vi "TF_Encoder2Position.vi"(2 "Counter Value":i32, 4 "Offset":dbl) -> (5 "Position [deg]":dbl format="%#_13g")   [LabVIEW 2019]
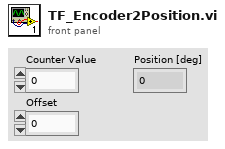
[diagram p1: front panel]
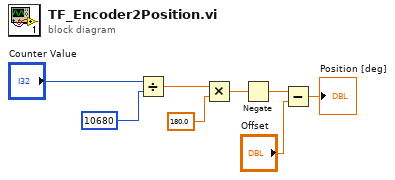
[diagram p0: block diagram]
diagram:
  n1 = Divide(x="Counter Value", y=10680) -> (x/y=w7:dbl)
  n2 = Multiply(x=w7, y=180.0) -> (x*y=w5:dbl)
  n3 = Negate(x=w5) -> (-x=w3:dbl)
  n4 = Subtract(x=w3, y="Offset") -> (x-y=→"Position [deg]":dbl)
